vi "Handle Error.vi"(8 "error in (no error)":errorcluster, 11 "LHW-GUI-Actor in":refnum<class "LHW-GUI-Actor.lvclass">) -> (0 "error out":errorcluster, 2 "stop actor?":bool=TRUE, 3 "LHW-GUI-Actor out":refnum<class "LHW-GUI-Actor.lvclass">)   [LabVIEW 2014, in "LHW-GUI.lvlib" / "LHW-GUI-Actor.lvclass"]
doc: "(<B>Filename</B>: Actor Framework.lvlib:Actor.lvclass:Handle Error.vi)\n\nDefines how the actor handles an error that occurred while processing a message. By default, this method does nothing except stop the actor."
uses:
  LHW-GUI-Actor.lvclass
  <vilib>/ActorFramework/Actor/Actor.lvclass
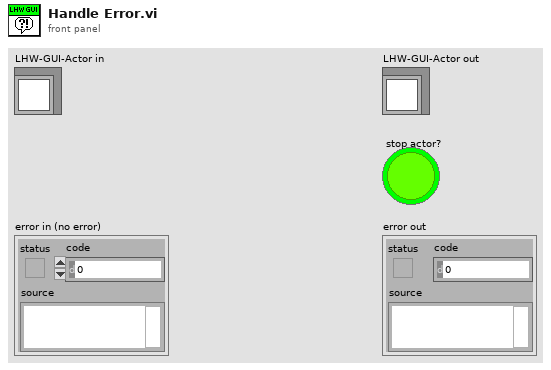
[diagram p1: front panel]
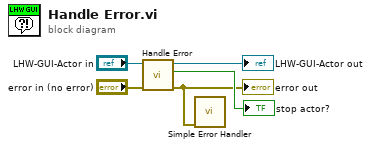
[diagram p0: block diagram]
diagram:
  n1 = call-parent "Handle Error.vi"("error in (no error)"="error in (no error)", "Actor in"="LHW-GUI-Actor in") -> ("error out"=w1:errorcluster, "stop actor?"=→"stop actor?":bool, "Actor out"=→"LHW-GUI-Actor out":refnum<class "LHW-GUI-Actor.lvclass">)  [unwired: 7 in]
  "error out" <- w1
  n2 = call <vilib>:"Simple Error Handler.vi"("error in (no error)"=w1) -> ()  [unwired: 4 in, 5 out]
